vi "Init.vi"(8 "error in (no error)":errorcluster, 10 "Channel":i16, 11 "EyeCalibration in":refnum<class "EyeCalibration.lvclass">) -> (0 "error out":errorcluster, 3 "EyeCalibration out":refnum<class "EyeCalibration.lvclass">)   [LabVIEW 2011, in "EyeCalibration.lvclass"]
uses:
  EyeCalibration.lvclass
  Trial Based Experiment Statechart/MatlabExperiment/MatlabExperiment.lvclass
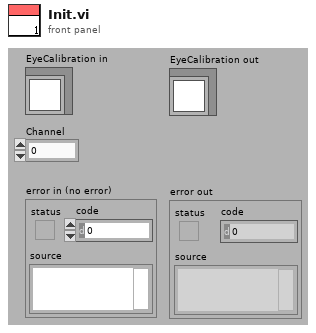
[diagram p1: front panel]
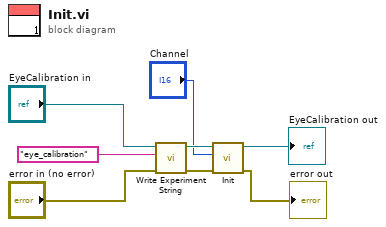
[diagram p0: block diagram]
diagram:
  n1 = call-dynamic "Write Experiment String.vi"("error in (no error)"="error in (no error)", "Experiment String"="eye_calibration", "TrialBasedExperiment in"="EyeCalibration in") -> ("error out"=w3:errorcluster, "TrialBasedExperiment out"=w6:refnum<class "EyeCalibration.lvclass">)  [unwired: 7 in]
  n2 = call-parent "Init.vi"("error in (no error)"=w3, "Channel"="Channel", "TrialBasedExperiment in"=w6) -> ("error out"=→"error out":errorcluster, "TrialBasedExperiment out"=→"EyeCalibration out":refnum<class "EyeCalibration.lvclass">)  [unwired: 7 in]
